vi "REG32.vi"(2 "D":u32 format="%x", 3 "R":bool, 4 "C":bool) -> (0 "~Q":u32=4294967295 format="%x", 1 "Q":u32 format="%x")   [LabVIEW 2019, in "Triggers.lvlib"]
uses:
  Triggers.lvlib
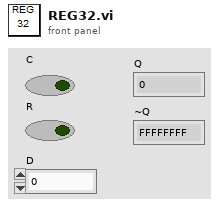
[diagram p1: front panel]
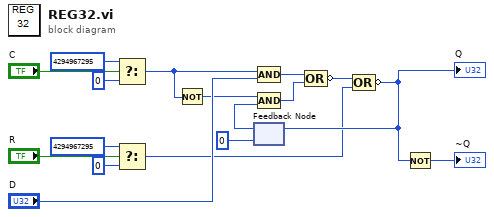
[diagram p0: block diagram]
diagram:
  n1 = Select(t=u32 4294967295, s="C", f=u32 0) -> (s? t:f=w5:u32)
  n2 = Select(t=u32 4294967295, s="R", f=u32 0) -> (s? t:f=w1:u32)
  n3 = Not(x=w5) -> (.not. x?=w15:u32)
  n4 = feedback #1(u32 0) -> (w14:u32)
  n5 = Compound Arithmetic op=AND(w5, "D") -> (w12:u32)
  n6 = Compound Arithmetic op=AND(w15, w14) -> (w11:u32)
  n7 = Compound Arithmetic op=OR(w12, w11) -> (invert w10:u32)
  n8 = Compound Arithmetic op=OR(w10, w1) -> (invert w9:u32)
  "Q" <- w9
  n9 = feedback-in #1(w9) -> ()
  n10 = Not(x=w9) -> (.not. x?=→"~Q":u32)
